vi "Set Position.vi"(8 "error in":errorcluster, 10 "Sequence Context In":refnum<k7>, 11 "VI Ref":refnum<vi>) -> (0 "error out":errorcluster)   [LabVIEW 2019, in "Diagonistics.lvlib"]
uses:
  Diagonistics.lvlib
  user32.dll
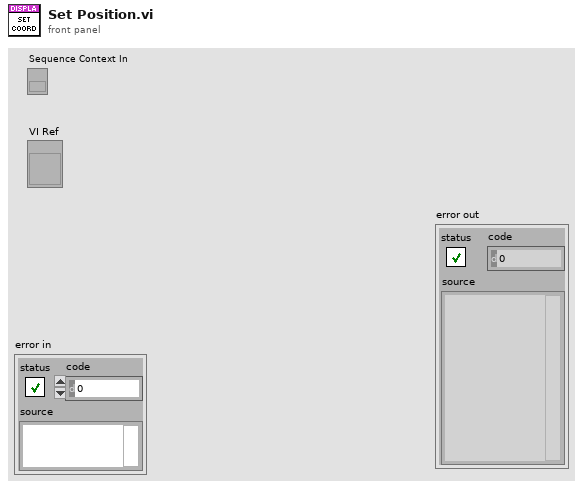
[diagram p1: front panel]
types:
  T1 = typedef "LVRectTypeDef.ctl" = cluster{"Left":i16, "Top":i16, "Right":i16, "Bottom":i16}
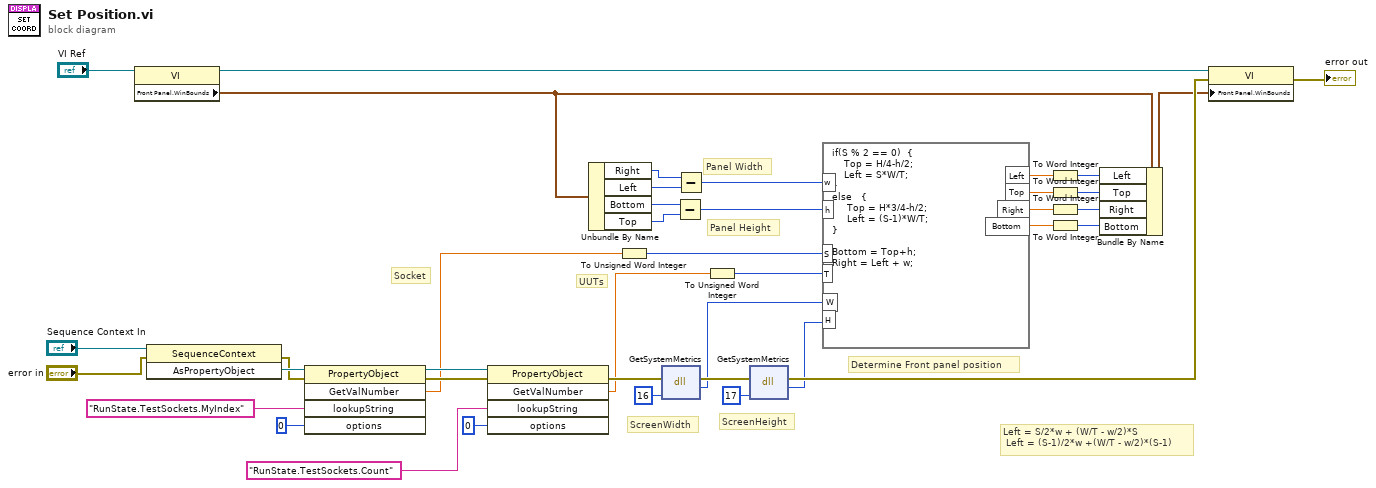
[diagram p0: block diagram]
diagram:
  # "Left = S/2*w + (W/T - w/2)*S\n Left = (S-1)/2*w +(W/T - w/2)*(S-1)"
  # "UUTs"
  # "Socket"
  # "Panel Height"
  # "Panel Width"
  # "Determine Front panel position"
  # "ScreenHeight"
  # "ScreenWidth"
  n1 = property class="VI"(reference="VI Ref") -> (reference out=w19:refnum<vi>, "Front Panel.WinBounds"=w31:T1)  [unwired: 1 in, 1 out]
  n2 = invoke class="SequenceContext" method="AsPropertyObject"(reference="Sequence Context In", error in="error in") -> (error out=w25:errorcluster, "AsPropertyObject"=w39:refnum<k7>)  [unwired: 1 in, 1 out]
  n3 = invoke class="PropertyObject" method="GetValNumber"(reference=w39, error in=w25, "lookupString"="RunState.TestSockets.MyIndex" ("Lookup String"), "options"=0) -> (reference out=w36:refnum<k7>, error out=w24:errorcluster, "GetValNumber"=w16:dbl)  [unwired: 1 in, 2 out]
  n4 = invoke class="PropertyObject" method="GetValNumber"(reference=w36, error in=w24, "lookupString"="RunState.TestSockets.Count" ("Lookup String"), "options"=0) -> (error out=w22:errorcluster, "GetValNumber"=w17:dbl)  [unwired: 1 in, 3 out]
  n5 = Unbundle By Name(w31) -> ("Right"=w30:i16, "Left"=w29:i16, "Bottom"=w28:i16, "Top"=w27:i16)
  n6 = To Unsigned Word Integer(number=w16) -> (unsigned 16bit integer=w12:u16)
  n7 = dll-call lib="user32.dll" fn="GetSystemMetrics"(error in=w22, "nIndex"=16) -> (error out=w23:errorcluster, "return type"=w14:i32)  [unwired: 3 in, 1 out]
  n8 = Subtract(x=w28, y=w27) -> (x-y=w10:i16)
  n9 = Subtract(x=w30, y=w29) -> (x-y=w11:i16)
  n10 = To Unsigned Word Integer(number=w17) -> (unsigned 16bit integer=w13:u16)
  n11 = dll-call lib="user32.dll" fn="GetSystemMetrics"(error in=w23, "nIndex"=17) -> (error out=w20:errorcluster, "return type"=w15:i32)  [unwired: 3 in, 1 out]
  n12 = formula code="if(S % 2 == 0)  {\n    Top = H/4-h/2;\n    Left = S*W/T;\n}\nelse   {\n     Top = H*3/4-h/2;\n     Left = (S-1)*W/T;\n}\n\nBottom = Top+h;\nRight = Left + w;"("S"=w12, "T"=w13, "W"=w14, "H"=w15, "w"=w11, "h"=w10) -> ("Left"=w6:dbl, "Top"=w9:dbl, "Right"=w8:dbl, "Bottom"=w7:dbl)
  n13 = To Word Integer(number=w6) -> (16bit integer=w1:i16)
  n14 = To Word Integer(number=w9) -> (16bit integer=w5:i16)
  n15 = To Word Integer(number=w8) -> (16bit integer=w4:i16)
  n16 = To Word Integer(number=w7) -> (16bit integer=w3:i16)
  n17 = Bundle By Name(cluster=w31, "Left"=w1, "Top"=w5, "Right"=w4, "Bottom"=w3) -> (w2:T1)
  n18 = property on="Property Node" class="VI"(reference=w19, error in=w20, "Front Panel.WinBounds"=w2) -> (error out=→"error out":errorcluster)  [unwired: 1 out]
